vi "Read Photon Counter Enqueuer.vi"(11 "Abstract Controller in":refnum<class "Abstract Controller.lvclass">) -> (2 "Actor Framework:Message Enqueuer":refnum<class "Message Enqueuer.lvclass">, 3 "Abstract Controller out":refnum<class "Abstract Controller.lvclass">)   [LabVIEW 2016, in "Controllers.lvlib" / "Abstract Controller.lvclass"]
uses:
  Abstract Controller.lvclass
  <vilib>/ActorFramework/Message Enqueuer/Message Enqueuer.lvclass
  Abstract Controller.lvclass/Abstract Controller.ctl
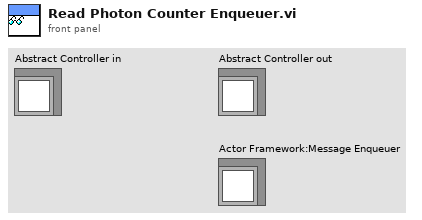
[diagram p1: front panel]
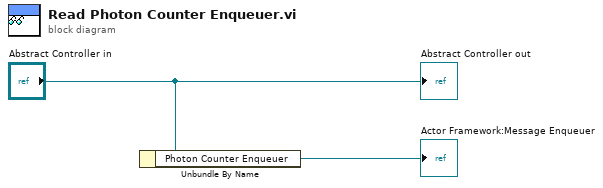
[diagram p0: block diagram]
diagram:
  n1 = Unbundle By Name("Abstract Controller in") -> ("Photon Counter Enqueuer"=→"Actor Framework:Message Enqueuer":refnum<class "Message Enqueuer.lvclass">)
  "Abstract Controller out" <- "Abstract Controller in"
